vi "ALU-5R.vi"(0 "a  2":bool, 1 "a  3":bool, 2 "a  4":bool, 3 "a  5":bool, 4 "B 5":bool, 5 "B 4":bool, 6 "B 3":bool, 7 "B 2":bool, 8 "a 1":bool, 9 "B 1":bool, 11 "C 1":bool, 13 "C 2":bool, 15 "C 3":bool, 17 "C 4":bool, 19 "C 5":bool) -> (20 "r 1":bool, 21 "r 2":bool, 22 "r 3":bool, 23 "r 4":bool, 24 "r 5":bool, 27 "S 1":bool)   [LabVIEW 2017]
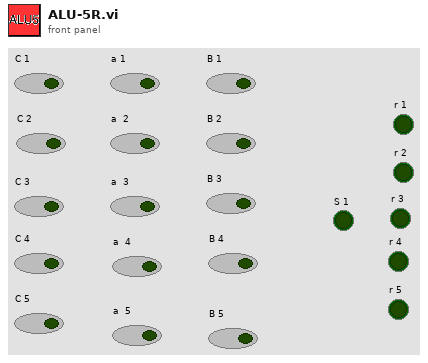
[diagram p1: front panel]
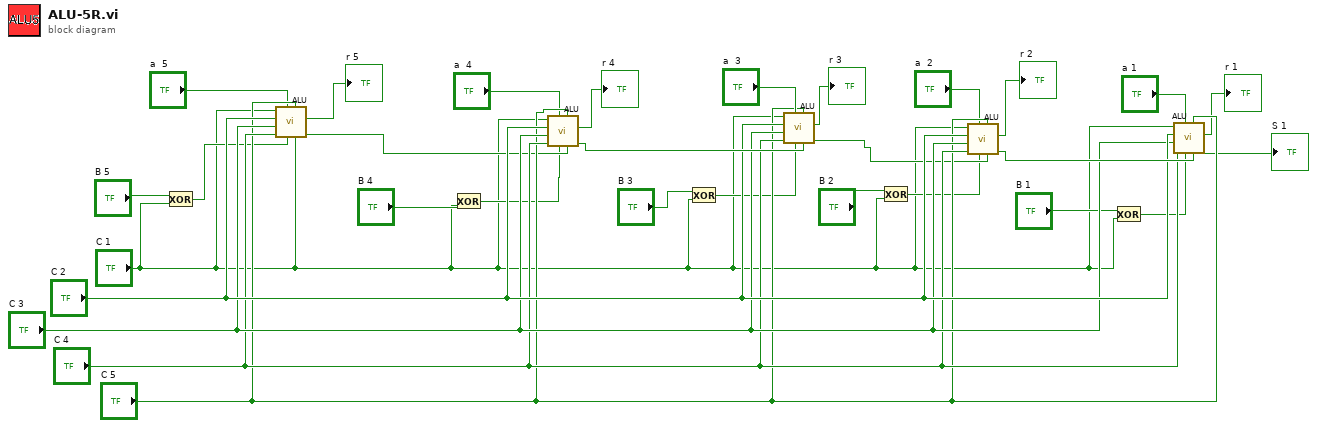
[diagram p0: block diagram]
diagram:
  n1 = Exclusive Or(1:"C 1", 2:"B 5") -> (0:w10:bool)
  n2 = call "ALU.vi"("S - 1"="C 1", "5"="C 5", 6:w10, 7:"a  5", "4"="C 4", "3"="C 3", "2"="C 2", "1"="C 1") -> ("cf"=w20:bool, "S"=→"r 5":bool)  [unwired: 2 in]
  n3 = Exclusive Or(1:"C 1", 2:"B 4") -> (0:w8:bool)
  n4 = call "ALU.vi"("S - 1"=w20, "5"="C 5", 6:w8, 7:"a  4", "4"="C 4", "3"="C 3", "2"="C 2", "1"="C 1") -> ("cf"=w30:bool, "S"=→"r 4":bool)  [unwired: 2 in]
  n5 = Exclusive Or(1:"C 1", 2:"B 3") -> (0:w6:bool)
  n6 = call "ALU.vi"("S - 1"=w30, "5"="C 5", 6:w6, 7:"a  3", "4"="C 4", "3"="C 3", "2"="C 2", "1"="C 1") -> ("cf"=w21:bool, "S"=→"r 3":bool)  [unwired: 2 in]
  n7 = Exclusive Or(1:"C 1", 2:"B 2") -> (0:w4:bool)
  n8 = call "ALU.vi"("S - 1"=w21, "5"="C 5", 6:w4, 7:"a  2", "4"="C 4", "3"="C 3", "2"="C 2", "1"="C 1") -> ("cf"=w27:bool, "S"=→"r 2":bool)  [unwired: 2 in]
  n9 = Exclusive Or(1:"C 1", 2:"B 1") -> (0:w2:bool)
  n10 = call "ALU.vi"("S - 1"=w27, "5"="C 5", 6:w2, 7:"a 1", "4"="C 4", "3"="C 3", "2"="C 2", "1"="C 1") -> ("cf"=→"S 1":bool, "S"=→"r 1":bool)  [unwired: 2 in]
